vi "XPath String Sub-Parser.vi"(3 "error in (no error)":errorcluster, 4 "XPath expression":string, 5 "XML String In":string) -> (0 "error out":errorcluster, 1 "Array of Results":string[](array[string]), 2 "XML String Out":string)   [LabVIEW 2013]
doc: "Use an XPath expression to search an XML string. An array containing all instances matching the search criteria will be returned.\n\nFor more information on XPath: http://www.w3schools.com/xpath/xpath_intro.asp"
uses:
  <vilib>/xml/Close Reference(Node).vi
  <vilib>/xml/NI_XML.lvlib
  <resource>/objmgr/DOMUserDefRef.rc
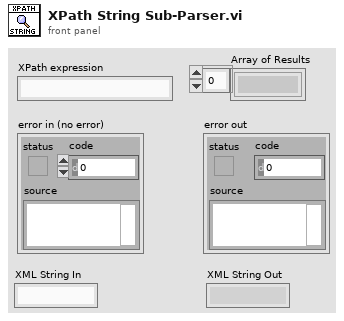
[diagram p1: front panel]
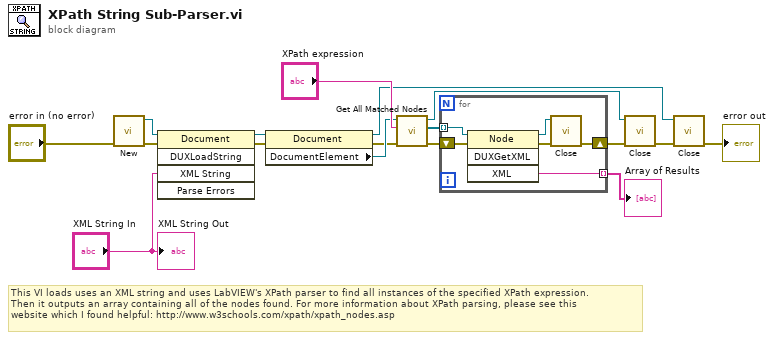
[diagram p0: block diagram]
diagram:
  # "This VI loads uses an XML string and uses LabVIEW's XPath parser to find all instances of the specified XPath expression. \nThen it outputs an array containing all of the nodes found. For more information about XPath parsing, please see this \nwebsite which I found helpful: http://www.w3schools.com/xpath/xpath_nodes.asp"
  n1 = call <vilib>:"New.vi"("error in (no error)"="error in (no error)") -> ("error out"=w1:errorcluster, "DOM document out"=w16:refnum<k20>)  [unwired: 7 in]
  n2 = invoke class="Document" method="DUXLoadString"(reference=w16, error in=w1, "XML String"="XML String In") -> (reference out=w15:refnum<k20>, error out=w14:errorcluster)  [unwired: 2 in, 3 out]
  n3 = property class="Document"(reference=w15, error in=w14) -> (reference out=w5:refnum<k20>, error out=w6:errorcluster, "DocumentElement"=w7:refnum<k20>)
  n4 = call <vilib>:"Get All Matched Nodes.vi"("error in (no error)"=w6, "XPath expression"="XPath expression", "node in"=w7) -> ("error out"=w11:errorcluster, "node result array"=w10:refnum<k20>[], "node out"=w4:refnum<k20>)  [unwired: 6 in]
  n5 = for {
    tunnel: w10 -> [w23] mode=indexing
    tunnel: [w22] -> w12 mode=indexing
    shift-right: [w18] -> w9
    shift-left: w11 -> [w21]
    n6 = invoke class="Node" method="DUXGetXML"(reference=w23, error in=w21) -> (reference out=w20:refnum<k20>, error out=w19:errorcluster, "XML"=w22:string)  [unwired: 2 in, 1 out]
    n7 = call-poly <vilib>:"Close.vi"("error in (no error)"=w19, "node"=w20) -> ("error out"=w18:errorcluster)  [unwired: 7 in]
  }
  "Array of Results" <- w12
  n8 = call-poly <vilib>:"Close.vi"("error in (no error)"=w9, "node"=w4) -> ("error out"=w8:errorcluster)  [unwired: 7 in]
  n9 = call-poly <vilib>:"Close.vi"("error in (no error)"=w8, "node"=w5) -> ("error out"=→"error out":errorcluster)  [unwired: 7 in]
  "XML String Out" <- "XML String In"
